vi "Main.vi"() -> ()   [LabVIEW 2020]
uses:
  <vilib>/DAQmx/read.llb/DAQmx Read (Digital 1D Bool 1Chan 1Samp).vi
  <vilib>/DAQmx/create/channels.llb/DAQmx Create Channel (DI-Digital Input).vi
  <vilib>/DAQmx/miscellaneous.llb/DAQmx Fill In Error Info.vi
  <vilib>/DAQmx/create/channels.llb/DAQmx Create Channel (AI-Voltage-Basic).vi
  <vilib>/DAQmx/create/channels.llb/DAQmx Create Channel (AO-Voltage-Basic).vi
  <vilib>/DAQmx/configure/timing.llb/DAQmx Timing (Sample Clock).vi
panel:
  in  "정지버튼":bool
  out "출력 문자열":string
  # "지진 감지 장치"
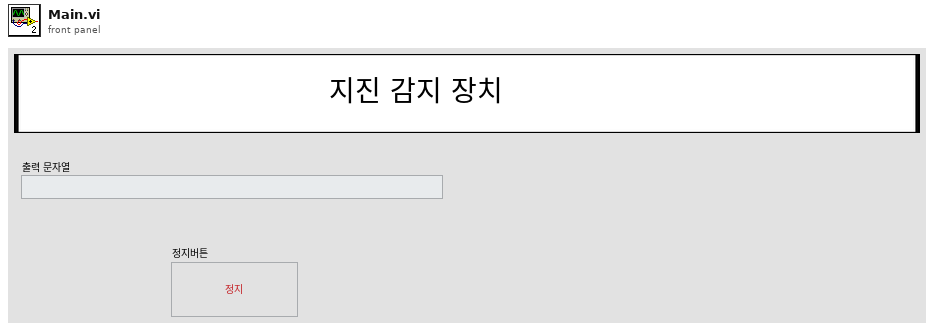
[diagram p1: front panel]
types:
  T1 = cluster{"출력 문자열":string, "알람 불리언":bool, "센서 불리언":bool[], "아날로그 출력 참조":refnum<k21>, "아날로그 입력 참조":refnum<k21>, "디지털 입력 참조":refnum<k21>, "감지시작 플레그":bool}
  T2 = typedef "지진계(열거형상수).ctl" = enum16{"초기화", "대기", "감지시작", "정지", "알림리셋"}
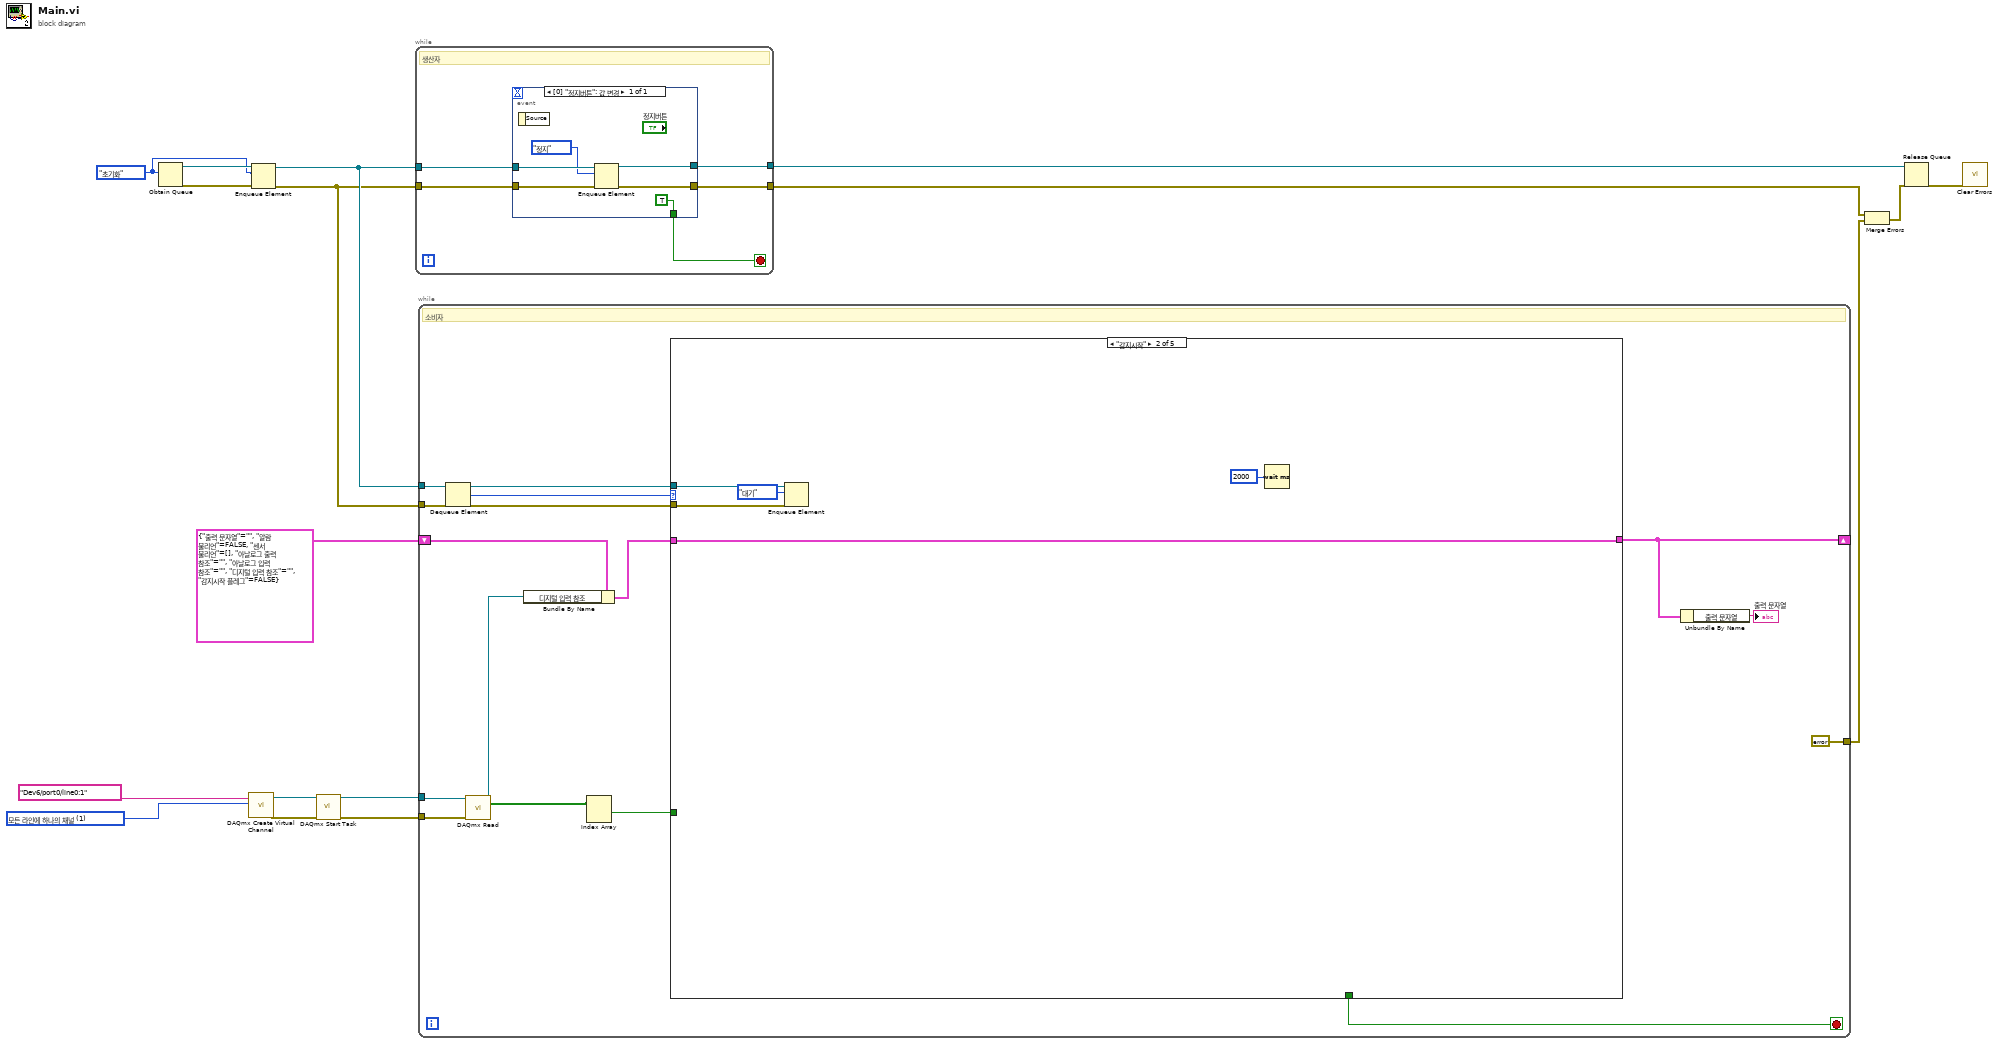
[diagram p0: block diagram]
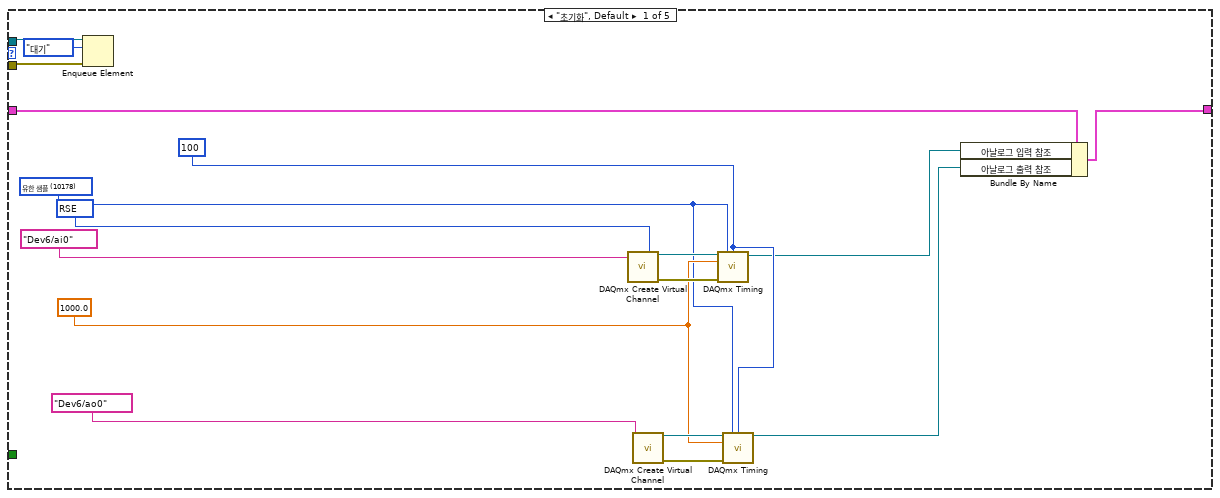
[diagram p2: hidden frame]
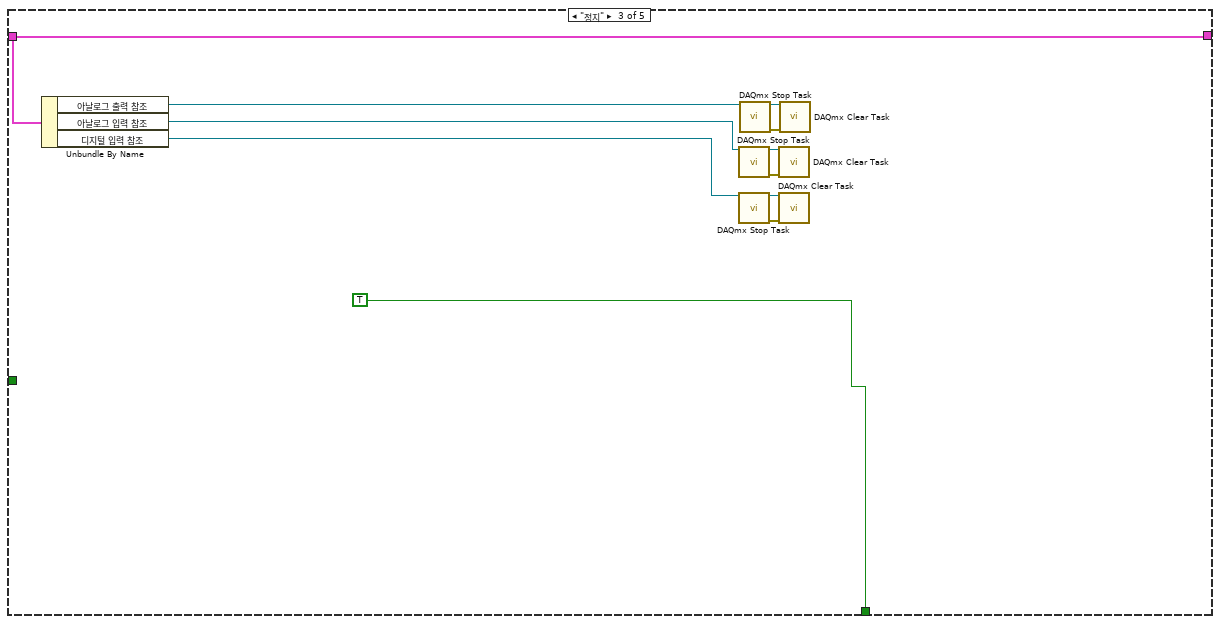
[diagram p3: hidden frame]
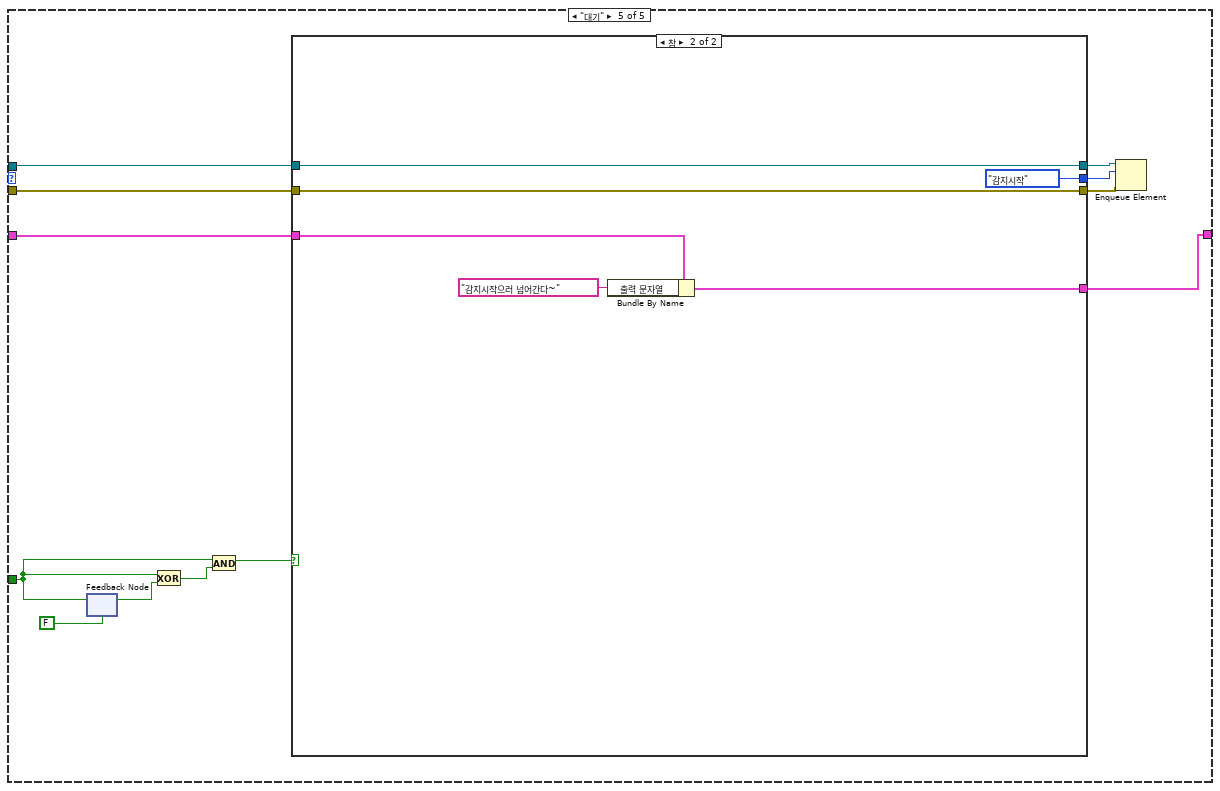
[diagram p5: hidden frame]
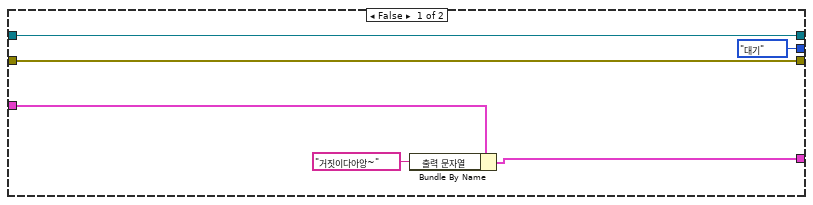
[diagram p6: hidden frame]
diagram:
  w2 = 1 items=["각 라인에 하나의 채널", "모든 라인에 하나의 채널"] ("line grouping")
  w8 = 지진계(열거형상수)."초기화" ("열거형")
  n1 = Obtain Queue(element data type=w8) -> (queue out=w16:refnum<queue>, error out=w17:errorcluster)  [unwired: 4 in, 1 out]
  n2 = call-poly <vilib>:"DAQmx Create Virtual Channel.vi"("lines"=tag "Dev6/port0/line0:1", "line grouping"=w2) -> ("task out"=w6:refnum<k21>, "error out"=w7:errorcluster)  [unwired: 12 in]
  n3 = Enqueue Element(queue=w16, element=w8, error in (no error)=w17) -> (queue out=w15:refnum<queue>, error out=w14:errorcluster)  [unwired: 1 in, 1 out]
  n4 = call <vilib>:"DAQmx Start Task.vi"("task/channels in"=w6, "error in"=w7) -> ("task out"=w5:refnum<k21>, "error out"=w4:errorcluster)  [unwired: 12 in]
  n5 = while {
    tunnel: w14 -> [w22]
    tunnel: w15 -> [w21]
    tunnel: [w20] -> w11
    tunnel: [w19] -> w13
    stop <- w18 stop-if-true
    # "생산자"
    n6 = event shown="[0] \"정지버튼\": 값 변경" {
      selector: _ -> [_]
      dyn-events: _ -> [_]
      timeout: _ -> [_]
      tunnel: w22 -> [w28]
      tunnel: w21 -> [w27]
      tunnel: [w26] -> w20
      tunnel: [w25] -> w19
      tunnel: [TRUE] -> w18
      event "정지버튼": Value Change {
        n7 = event-data() -> ()  [unwired: 1 in, 1 out]
        n8 = Enqueue Element(queue=w27, element=지진계(열거형상수)."정지" ("열거형"), error in (no error)=w28) -> (queue out=w25:refnum<queue>, error out=w26:errorcluster)  [unwired: 1 in, 1 out]
      }
    }
  }
  n9 = while {
    tunnel: w15 -> [w44]
    tunnel: w14 -> [w43]
    tunnel: [errorcluster {"status"=FALSE, "code"=0, "source"=""} ("에러 상수")] -> w10
    tunnel: w5 -> [w36]
    tunnel: w4 -> [w40]
    shift-right: [w34] -> _
    shift-left: T1 {"출력 문자열"="", "알람 불리언"=FALSE, "센서 불리언"=[], "아날로그 출력 참조"="", "아날로그 입력 참조"="", "디지털 입력 참조"="", "감지시작 플레그"=FALSE} -> [w37]
    stop <- w41 stop-if-true
    # "소비자"
    n10 = Dequeue Element(queue=w44, error in (no error)=w43) -> (queue out=w39:refnum<queue>, element=w31:T2, error out=w38:errorcluster)  [unwired: 1 in, 1 out]
    n11 = call-poly <vilib>:"DAQmx Read.vi"("task/channels in"=w36, "error in"=w40) -> ("task out"=w32:refnum<k21>, "data"=w30:bool[])  [unwired: 11 in, 1 out]
    n12 = Bundle By Name(cluster=w37, "디지털 입력 참조"=w32) -> (w35:T1)
    n13 = Index Array(array=w30) -> (element #1=w29:bool)  [unwired: 2 in, 1 out]
    n14 = case shown="\"감지시작\"" w31 {
      tunnel: [_ _ TRUE _ _] -> w41
      tunnel: w39 -> [w49 w66 _ _ w85]
      tunnel: w38 -> [w48 w65 _ _ w84]
      tunnel: w35 -> [w52 w63 w76 w78 w83]
      tunnel: [w50 w63 w76 w78 w82] -> w34
      tunnel: w29 -> [_ _ _ _ w87]
      frame "초기화", Default {
        w46 = 100 ("samples per channel")
        w53 = 10178 items=["유한 샘플"=10178, "연속 샘플"=10123, "하드웨어 타이밍에 의한 단일 포인트"=12522] ("sample mode")
        w54 = 1000.0 ("rate")
        w60 = 10083 items=["기본"=-1, "RSE"=10083, "NRSE"=10078, "차동"=10106, "유사 차동"=12529] ("input terminal configuration")
        n15 = Enqueue Element(queue=w49, element=지진계(열거형상수)."대기" ("원소"), error in (no error)=w48) -> ()  [unwired: 1 in, 3 out]
        n16 = call-poly <vilib>:"DAQmx Create Virtual Channel.vi"("input terminal configuration"=w60, "physical channels"=tag "Dev6/ai0") -> ("task out"=w59:refnum<k21>, "error out"=w58:errorcluster)  [unwired: 12 in]
        n17 = call-poly <vilib>:"DAQmx Create Virtual Channel.vi"("physical channels"=tag "Dev6/ao0") -> ("task out"=w56:refnum<k21>, "error out"=w57:errorcluster)  [unwired: 13 in]
        n18 = call-poly <vilib>:"DAQmx Timing.vi"("task/channels in"=w59, "sample mode"=w53, "samples per channel"=w46, "rate"=w54, "error in"=w58) -> ("task out"=w45:refnum<k21>)  [unwired: 9 in, 1 out]
        n19 = call-poly <vilib>:"DAQmx Timing.vi"("task/channels in"=w56, "sample mode"=w53, "samples per channel"=w46, "rate"=w54, "error in"=w57) -> ("task out"=w51:refnum<k21>)  [unwired: 9 in, 1 out]
        n20 = Bundle By Name(cluster=w52, "아날로그 입력 참조"=w45, "아날로그 출력 참조"=w51) -> (w50:T1)
      }
      frame "감지시작" {
        n21 = Enqueue Element(queue=w66, element=지진계(열거형상수)."대기" ("원소"), error in (no error)=w65) -> ()  [unwired: 1 in, 3 out]
        n22 = Wait (ms)(milliseconds to wait=u32 2000 ("대기 시간 (ms)")) -> ()  [unwired: 1 out]
      }
      frame "정지" {
        n23 = Unbundle By Name(w76) -> ("아날로그 출력 참조"=w69:refnum<k21>, "아날로그 입력 참조"=w68:refnum<k21>, "디지털 입력 참조"=w67:refnum<k21>)
        n24 = call <vilib>:"DAQmx Stop Task.vi"("task/channels in"=w68) -> ("task out"=w72:refnum<k21>, "error out"=w73:errorcluster)  [unwired: 13 in]
        n25 = call <vilib>:"DAQmx Stop Task.vi"("task/channels in"=w67) -> ("task out"=w71:refnum<k21>, "error out"=w70:errorcluster)  [unwired: 13 in]
        n26 = call <vilib>:"DAQmx Stop Task.vi"("task/channels in"=w69) -> ("task out"=w75:refnum<k21>, "error out"=w74:errorcluster)  [unwired: 13 in]
        n27 = call <vilib>:"DAQmx Clear Task.vi"("task in"=w72, "error in"=w73) -> ()  [unwired: 13 in, 1 out]
        n28 = call <vilib>:"DAQmx Clear Task.vi"("task in"=w71, "error in"=w70) -> ()  [unwired: 13 in, 1 out]
        n29 = call <vilib>:"DAQmx Clear Task.vi"("task in"=w75, "error in"=w74) -> ()  [unwired: 13 in, 1 out]
      }
      frame "알림리셋" {
      }
      frame "대기" {
        n30 = feedback-in #1(w87) -> ()
        n31 = feedback #1(FALSE) -> (w89:bool)
        n32 = Exclusive Or(1:w89, 2:w87) -> (0:w88:bool)
        n33 = And(x=w87, y=w88) -> (x .and. y?=w86:bool)
        n34 = case shown="참" w86 {
          tunnel: w85 -> [w96 w99]
          tunnel: w84 -> [w95 w98]
          tunnel: w83 -> [w93 w102]
          tunnel: [w92 w101] -> w82
          tunnel: [w96 w99] -> w81
          tunnel: [w95 w98] -> w80
          tunnel: [지진계(열거형상수)."대기" ("원소") 지진계(열거형상수)."감지시작" ("원소")] -> w79
          frame False {
            n35 = Bundle By Name(cluster=w93, "출력 문자열"="거짓이다아앙~") -> (w92:T1)
          }
          frame True {
            n36 = Bundle By Name(cluster=w102, "출력 문자열"="감지시작으러 넘어간다~") -> (w101:T1)
          }
        }
        n37 = Enqueue Element(queue=w81, element=w79, error in (no error)=w80) -> ()  [unwired: 1 in, 3 out]
      }
    }
    n38 = Unbundle By Name(w34) -> ("출력 문자열"=→"출력 문자열":string)
  }
  n39 = Merge Errors(w11, w10) -> (w9:errorcluster)
  n40 = Release Queue(queue=w13, error in (no error)=w9) -> (error out=w12:errorcluster)  [unwired: 1 in, 2 out]
  n41 = call <vilib>:"Clear Errors.vi"("error in (no error)"=w12) -> ()  [unwired: 5 in, 2 out]
